vi "CAMERA.vi"() -> ()   [LabVIEW 2015]
uses:
  Controls/HID Data.ctl
  <vilib>/userdefined/High Color/IMAQdx.ctl
  <vilib>/vision/Image Controls.llb/IMAQ Image.ctl
  Controls/HID State.ctl
  Controls/FGV_Options.ctl
  <vilib>/nisyscfg/Close (System).vi
  <vilib>/nisyscfg/nisyscfg.lvlib
  <resource>/objmgr/motionsysapi.rc
panel:
  out "TXT_001":string
  in  "Available Cameras":i32(listbox)=-1
  in  "BOOL_004":bool
  in  "BOOL_003":bool
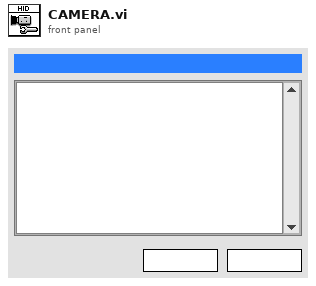
[diagram p1: front panel]
types:
  T1 = typedef "FGV_Options.ctl" = enum16{"Read from File", "Write to File", "Get", "Set"}
  T2 = typedef "HID Data.ctl" = cluster{"IMAQdx Session":T3, "Resampled Image":T4, "Low Level Grab":T4, "X Resolution":i32, "Y Resolution":i32, "Image Threshold":u8, "Reset Value":i32, "FIFO Timer":u16, "Row Timer":u32, "Memory Writer Timer":u8, "Color":enum16{"Green", "Blue", "Red", "White", "Pink", "Yellow", "Turquoise", "Black"}, "Top":bool[][], "Bottom":bool[][], "Timeout (ms)":i32, "Menu Tag":string, "Color Background":enum16{"Green", "Blue", "Red", "White", "Pink", "Yellow", "Turquoise", "Black"}, "FPGA VI Reference":refnum<k20>, "Next Steps":T5[], "Turn off LED Matrix":bool, "FPGA Alias":string, "FPGA Bitfile":path, "Localized Texts":cluster{"Status Text":cluster{"Status Text Table":string[], "Status Text Index":i32}, "Controls":cluster{"Control Text Table":string[], "Control Text Index":i32}, "Titles":cluster{"Titles Text Table":string[], "Titles Text Index":i32}}, "Language":u16}
  T3 = typedef "IMAQdx.ctl" = refnum<k21>
  T4 = typedef "IMAQ Image.ctl" = refnum<image>
  T5 = typedef "HID State.ctl" = enum16{"Initialize", "Set FPGA Parametes", "Set Camera Parameters", "Set LED Matrix Parameters", "Initialize FPGA Interface", "Initialize Camera", "Start FPGA VI", "Start Camera", "Wait for Event", "Update UI", "Acquire", "Process Image", "Get Boolean Arrays", "Send to FPGA", "Menu Pop-Up", "Menu Actions", "Handle Errors", "Close Camera", "Close FPGA", "Stop", "Exit"}
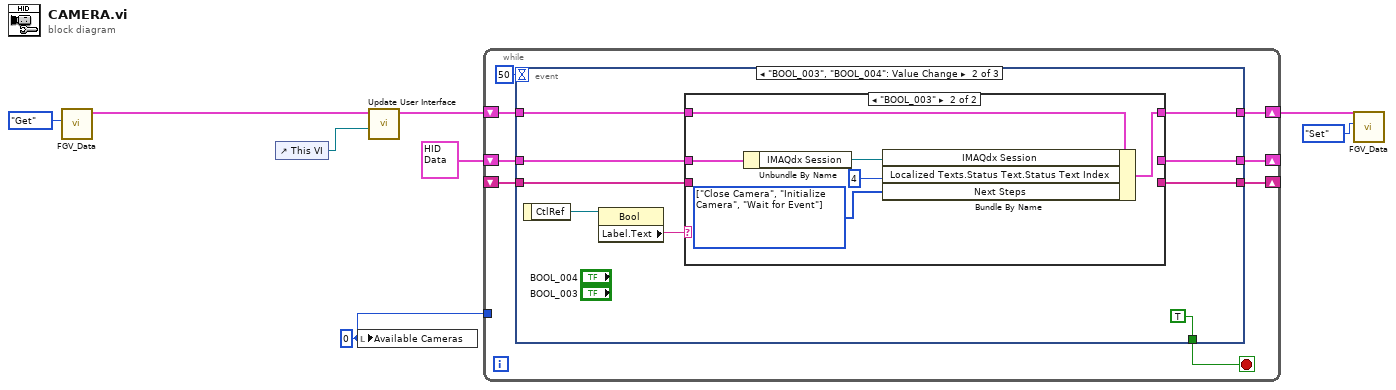
[diagram p0: block diagram]
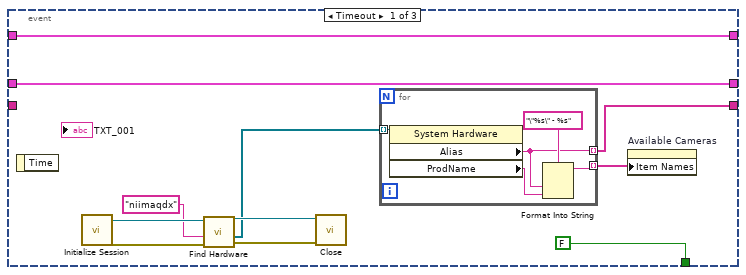
[diagram p2: hidden frame]
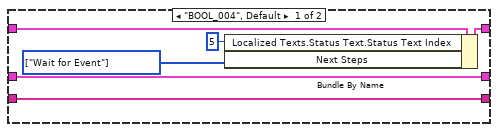
[diagram p3: hidden frame]
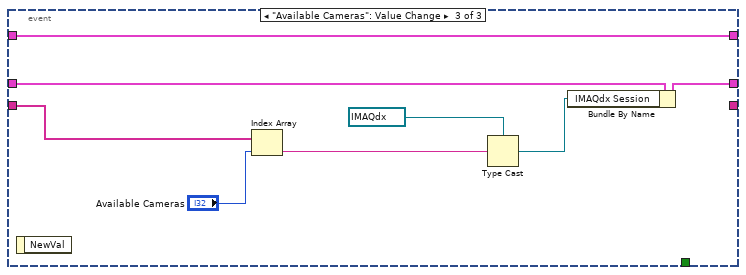
[diagram p4: hidden frame]
diagram:
  w7 = 0 ("Available Cameras")
  n1 = call "FGV_Data.vi"("Option"=FGV_Options."Get") -> ("Data Out"=w2:T2)  [unwired: 9 in, 1 out]
  n2 = control-ref of="This VI"() -> (w3:refnum<vi>)
  n3 = local write "Available Cameras"(w7) -> ()
  n4 = call "Update User Interface.vi"("VI Refnum"=w3, "Data In"=w2) -> ("Data Out"=w1:T2)  [unwired: 8 in, 1 out]
  n5 = while {
    shift-right: [w16] -> w4
    shift-left: w1 -> [w15]
    shift-right: [w12] -> _
    shift-left: T2 {"IMAQdx Session"="", "Resampled Image"=refnum, "Low Level Grab"=refnum, "X Resolution"=0, "Y Resolution"=0, "Image Threshold"=0, "Reset Value"=0, "FIFO Timer"=0, "Row Timer"=0, "Memory Writer Timer"=0, "Color"=enum."Red", "Top"=array32x96[3072 elements], "Bottom"=array32x96[3072 elements], "Timeout (ms)"=0, "Menu Tag"="", "Color Background"=enum."White", "FPGA VI Reference"=refnum, "Next Steps"=[], "Turn off LED Matrix"=FALSE, "FPGA Alias"="", "FPGA Bitfile"=path "", "Localized Texts"={"Status Text"={"Status Text Table"=[], "Status Text Index"=0}, "Controls"={"Control Text Table"=[], "Control Text Index"=0}, "Titles"={"Titles Text Table"=[], "Titles Text Index"=0}}, "Language"=0} ("Data In TMP") -> [w13]
    shift-right: [w10] -> _
    shift-left: _ -> [w9]
    tunnel: w7 -> [_]
    stop <- w14 stop-if-true
    n6 = event shown="[1] \"BOOL_003\", \"BOOL_004\": Value Change" {
      selector: _ -> [_ _ _]
      dyn-events: _ -> [_ _ _]
      timeout: 50 -> [_ _ _]
      tunnel: [w27 w38 w61] -> w16
      tunnel: w15 -> [w27 w39 w61]
      tunnel: [FALSE TRUE _] -> w14
      tunnel: w13 -> [w26 w36 w60]
      tunnel: [w26 w33 w55] -> w12
      tunnel: [w17 w34 _] -> w10
      tunnel: w9 -> [_ w35 w56]
      event Timeout {
        n7 = event-data() -> ()  [unwired: 1 in, 1 out]
        n8 = call <vilib>:"Initialize Session.vi"() -> ("error out"=w24:errorcluster, "Session out"=w22:refnum<k21>)  [unwired: 10 in]
        n9 = call <vilib>:"Find Hardware.vi"("error in (no error)"=w24, "Experts"="niimaqdx", "Session in"=w22) -> ("error out"=w23:errorcluster, "Resources out"=w19:refnum<k20>[], "Session out"=w21:refnum<k21>)  [unwired: 5 in, 1 out]
        n10 = call-poly <vilib>:"Close.vi"("error in (no error)"=w23, "Session in"=w21) -> ()  [unwired: 9 in, 1 out]
        n11 = for {
          tunnel: w19 -> [w32] mode=indexing
          tunnel: [w28] -> w18 mode=indexing
          tunnel: [w30] -> w17 mode=indexing
          n12 = property class="System Hardware"(reference=w32) -> ("Alias"=w30:string, "ProdName"=w29:string)  [unwired: 1 in, 2 out]
          n13 = Format Into String(format string="\"%s\" - %s", w30, w29) -> (resulting string=w28:string)  [unwired: 2 in, 1 out]
        }
        n14 = property on="Available Cameras" class="LstBox (strict)"("Item Names"=w18) -> ()  [unwired: 2 in, 2 out]
      }
      event "BOOL_003", "BOOL_004": Value Change {
        n15 = event-data() -> ("CtlRef"=w40:refnum<vi>)  [unwired: 1 in]
        n16 = property class="Bool"(reference=w40) -> ("Label.Text"=w37:string)  [unwired: 1 in, 2 out]
        n17 = case shown="\"BOOL_003\"" w37 {
          tunnel: w39 -> [w47 w53]
          tunnel: [w46 w52] -> w38
          tunnel: w36 -> [w44 w51]
          tunnel: w35 -> [w45 _]
          tunnel: [w45 _] -> w34
          tunnel: [w44 _] -> w33
          frame "BOOL_004", Default {
            w43 = T5[] [enum."Wait for Event"] items=["Initialize", "Set FPGA Parametes", "Set Camera Parameters", "Set LED Matrix Parameters", "Initialize FPGA Interface", "Initialize Camera", "Start FPGA VI", "Start Camera", "Wait for Event", "Update UI", "Acquire", "Process Image", "Get Boolean Arrays", "Send to FPGA", "Menu Pop-Up", "Menu Actions", "Handle Errors", "Close Camera", "Close FPGA", "Stop", "Exit"] ("Array")
            n18 = Bundle By Name(cluster=w47, "Localized Texts.Status Text.Status Text Index"=5 ("Status"), "Next Steps"=w43) -> (w46:T2)
          }
          frame "BOOL_003" {
            w49 = T5[] [enum."Close Camera", enum."Initialize Camera", enum."Wait for Event"] items=["Initialize", "Set FPGA Parametes", "Set Camera Parameters", "Set LED Matrix Parameters", "Initialize FPGA Interface", "Initialize Camera", "Start FPGA VI", "Start Camera", "Wait for Event", "Update UI", "Acquire", "Process Image", "Get Boolean Arrays", "Send to FPGA", "Menu Pop-Up", "Menu Actions", "Handle Errors", "Close Camera", "Close FPGA", "Stop", "Exit"] ("Array")
            n19 = Unbundle By Name(w51) -> ("IMAQdx Session"=w50:T3)
            n20 = Bundle By Name(cluster=w53, "IMAQdx Session"=w50, "Localized Texts.Status Text.Status Text Index"=4 ("Status"), "Next Steps"=w49) -> (w52:T2)
          }
        }
      }
      event "Available Cameras": Value Change {
        n21 = event-data() -> ()  [unwired: 1 in, 1 out]
        n22 = Index Array(array=w56, index="Available Cameras") -> (element=w59:string)
        n23 = Type Cast(type=T3 "cam0" ("IMAQdx Session"), x=w59) -> (*(type *) &x=w54:T3)
        n24 = Bundle By Name(cluster=w60, "IMAQdx Session"=w54) -> (w55:T2)
      }
    }
  }
  n25 = call "FGV_Data.vi"("Option"=FGV_Options."Set", "Data In"=w4) -> ()  [unwired: 8 in, 2 out]
